vi "Find Hynix Spec.vi"(8 "error in":errorcluster) -> (0 "error out":errorcluster)   [LabVIEW 2020]
uses:
  Controls/Comm_Hynix Spec.ctl
  Controls/Cmd_File path.ctl
  <vilib>/Utility/sysdir.llb/System Directory Type.ctl
  Controls/Cmd_File Type.ctl
  <vilib>/Utility/NIReport.llb/Report Type.ctl
  Public/Polymorph/ini Ctrl_Str.vi
  Public/Polymorph/ini Ctrl_Var.vi
  <vilib>/security/Message Digest/API/Instances/File/SHA-256 File Checksum.vi
  <vilib>/addons/_office/excel.llb/Excel Get Data ([str]).vi
  <vilib>/Utility/NIReport.llb/NI_report.lvclass
  <vilib>/Utility/NIReport.llb/NI_ReportGenerationCore.lvlib
  <vilib>/addons/_office/NI_ReportGenerationToolkit.lvlib
  <vilib>/Utility/NIReport.llb/Excel/NI_Excel.lvclass
  <vilib>/security/Message Digest/API/NI_Message Digest API.lvlib
  <vilib>/addons/database/NI_Database_API.lvlib
panel:
  out "Status":string
  in  "파일 경로":path
  in  "팀":bool
  in  "모델":bool
  in  "제조사":bool
  in  "기기명":bool
  in  "Team SPEC":i32(listbox)
  in  "확인 버튼":bool
  in  "프로세스 정지 버튼":bool
  out "SPEC":string[][](table)
  in  "등록번호":string
  out "digest":string caption="요약"
  out "data":string[][](array[string])
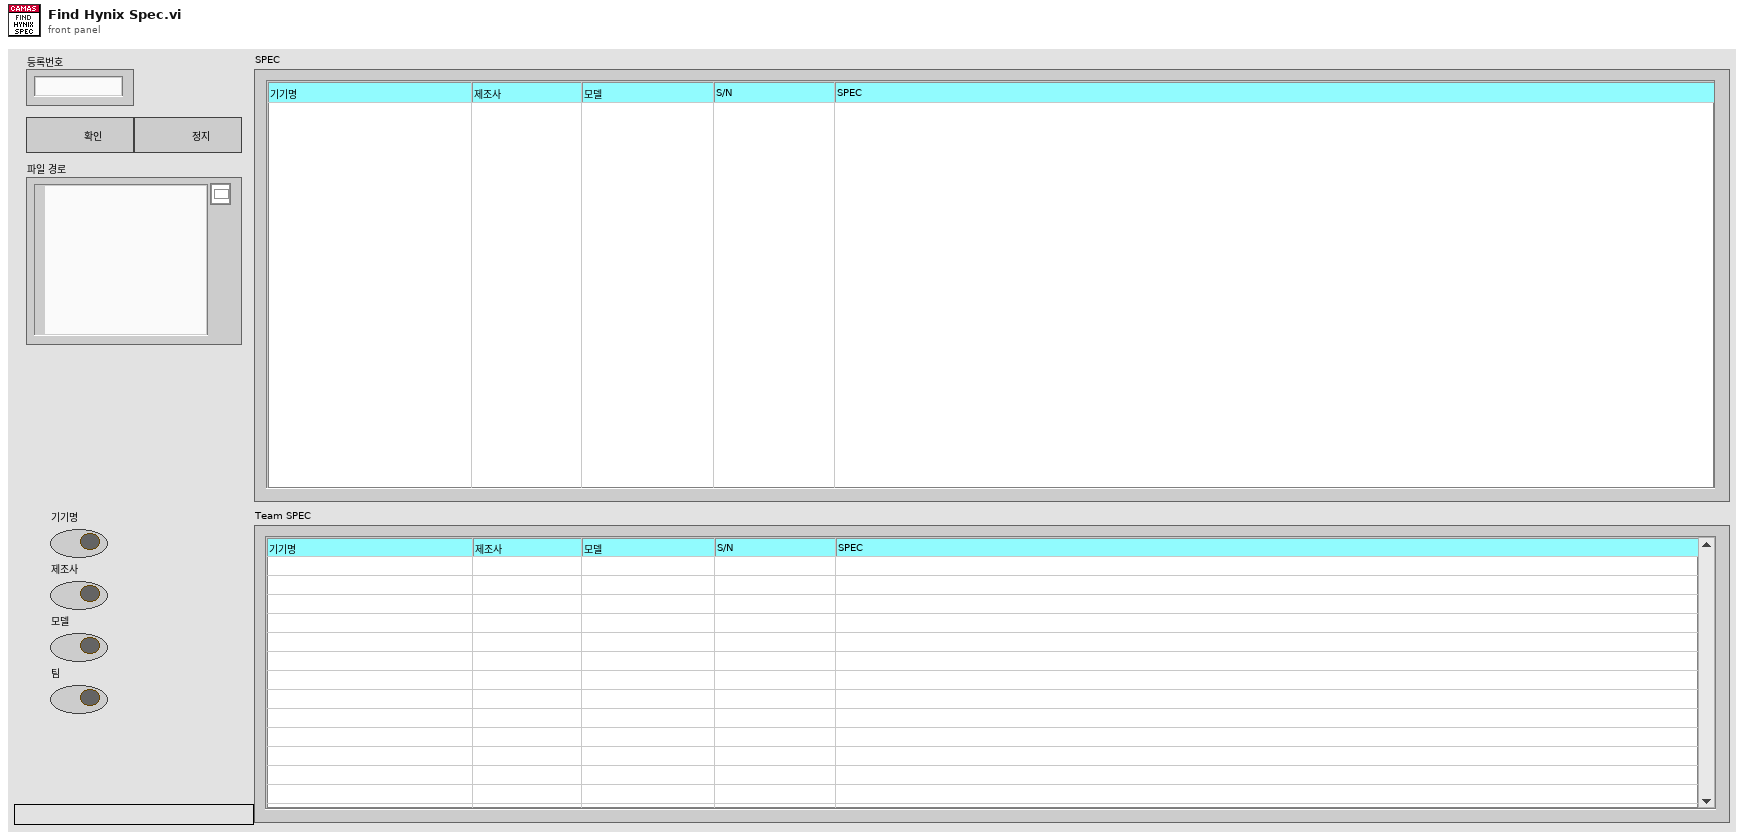
[diagram p1: front panel]
types:
  T1 = typedef "Comm_Hynix Spec.ctl" = enum16{"Initialize", "event", "File Open", "Find Spec", "Team Spec Open", "Error", "Exit"}
  T2 = typedef "Cmd_File Type.ctl" = enum16{"엑셀", "엑셀(2003)", "텍스트", "설정", "2진", "VI", "CSV", "LOG", "폴더"}
  T3 = typedef "Cmd_File path.ctl" = enum16{"에러로그", "데이터파일경로", "성적서원본", "지난성적서", "Data Files", "경로생성", "Updater", "Template", "설정파일경로", "FTP Upload", "Update 경로", "어플리케이션"}
  T4 = typedef "System Directory Type.ctl" = i32
  T5 = enum16{"open", "replace", "create", "open or create", "replace or create", "replace or create with confirmation"}
  T6 = typedef "NI_ReportGenerationCore.lvlib/Report Type.ctl" = enum16{"HTML", "Word", "Excel"}
  T7 = enum16{"maximized", "minimized", "normal", "no change"}
  T8 = cluster{"position (excel)":cluster{"row":i32, "column":i32}, "name (excel)":string, "bookmark (word)":string}
  T9 = typedef "NI_Database_API.lvlib/Conn ObjectReference.ctl" = refnum<k1>
  T10 = enum32{"invalid app kind", "Development System", "Run Time System", "Student Edition", "Embedded LabVIEW", "Evaluation", "Custom"}
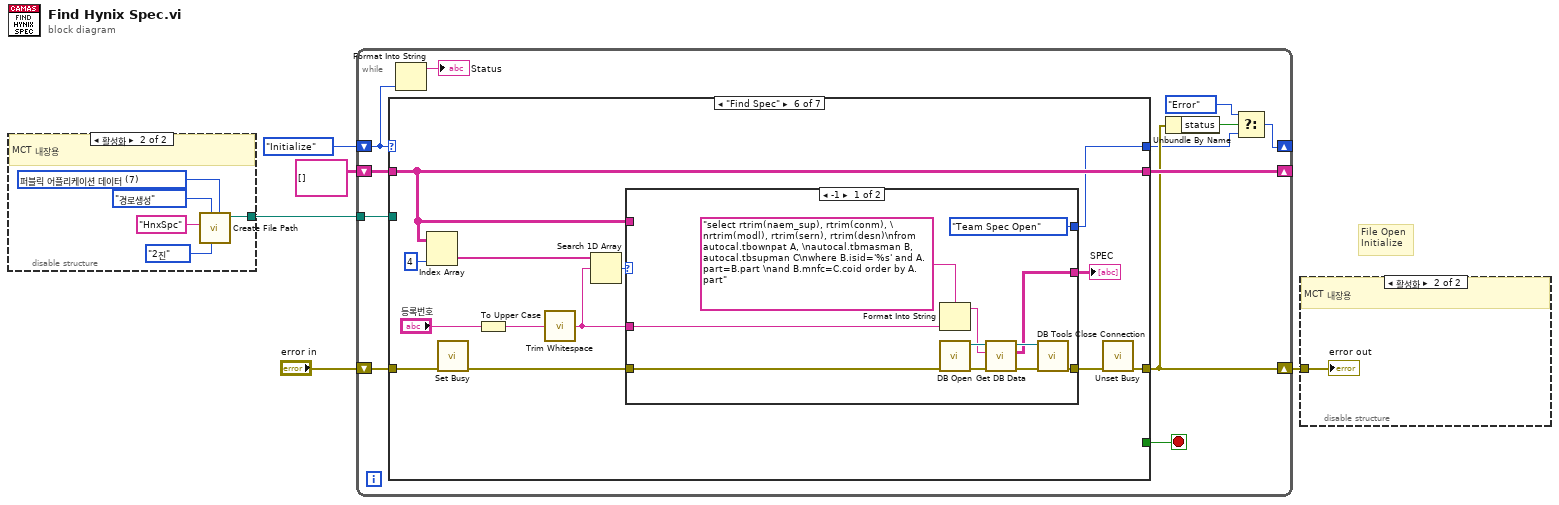
[diagram p0: block diagram]
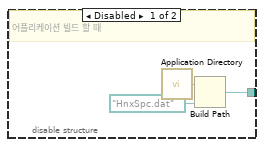
[diagram p2: hidden frame]
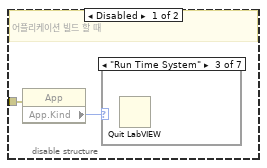
[diagram p3: hidden frame]
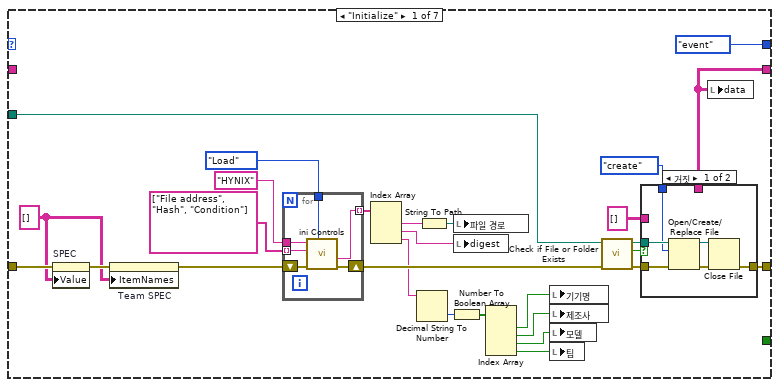
[diagram p10: hidden frame]
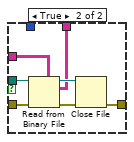
[diagram p11: hidden frame]
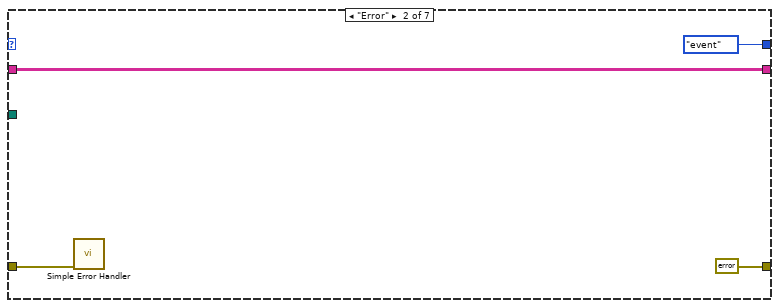
[diagram p12: hidden frame]
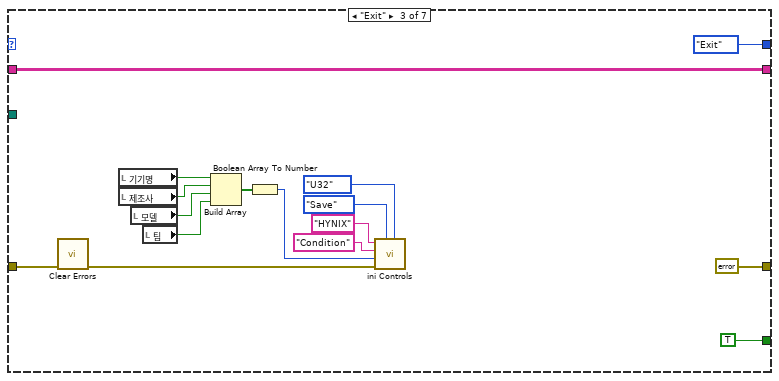
[diagram p13: hidden frame]
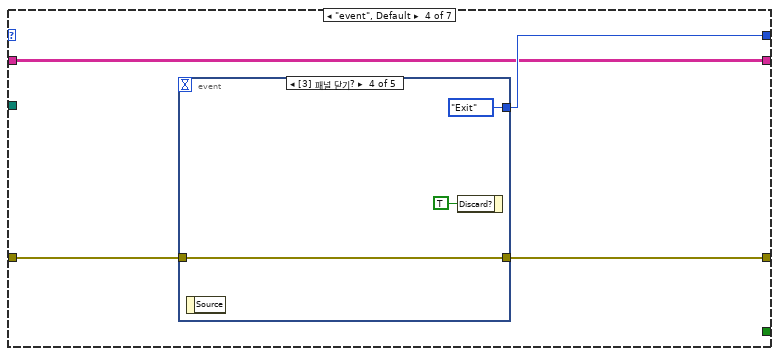
[diagram p14: hidden frame]
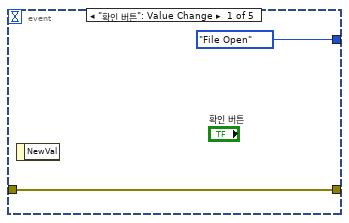
[diagram p15: hidden frame]
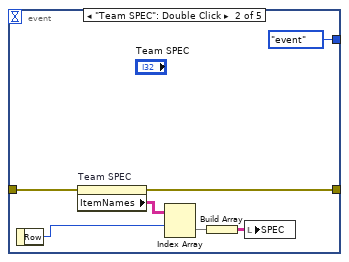
[diagram p16: hidden frame]
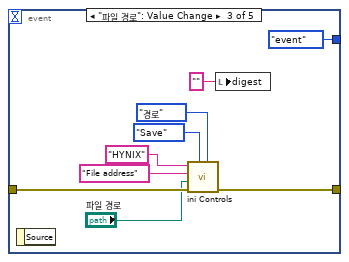
[diagram p17: hidden frame]
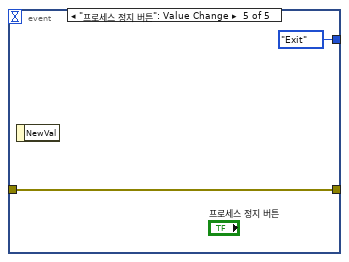
[diagram p18: hidden frame]
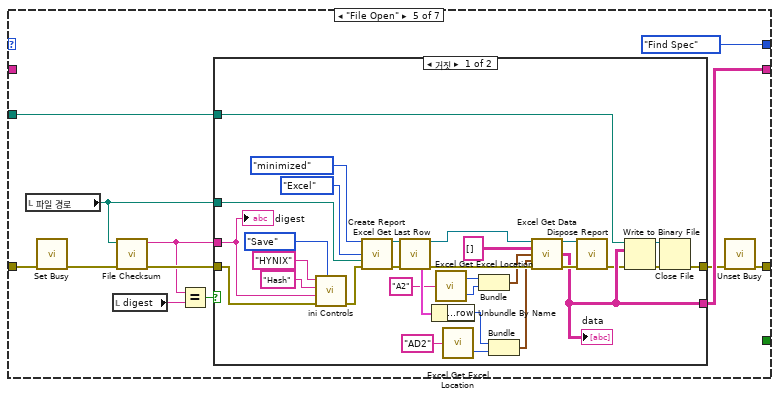
[diagram p19: hidden frame]
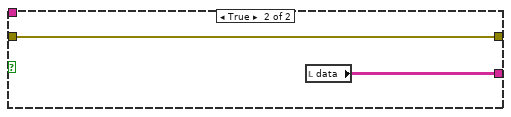
[diagram p20: hidden frame]
diagram:
  # "File Open\nInitialize"
  n1 = disable-structure shown="활성화" {
    disable-tunnel: [w6 w13] -> w1
    frame Disabled {
      # "어플리케이션 빌드 할 때"
      n2 = call <vilib>:"Application Directory.vi"() -> ("Application Directory"=w8:path)
      n3 = Build Path(base path=w8, name or relative path=path "HnxSpc.dat" ("이름 또는 상대 경로")) -> (appended path=w6:path)
    }
    frame Enabled {
      w11 = T4 7 items=["사용자 홈"=0, "사용자 데스크탑"=1, "사용자 문서"=2, "사용자 어플리케이션 데이터"=3, "사용자 환경"=4, "사용자 임시"=5, "퍼블릭 문서"=6, "퍼블릭 어플리케이션 데이터"=7, "퍼블릭 환경"=8, "퍼블릭 캐시"=13, "시스템 코어 라이브러리"=9, "시스템 설치된 라이브러리"=10, "어플리케이션 파일"=11, "부팅 볼륨 루트"=12] ("system directory type")
      # "MCT 내장용"
      n4 = call "Create File Path.vi"("system directory type"=w11, "파일타입"=Cmd_File_Type."2진", "항목"=Cmd_File_path."경로생성", "문자열 in"="HnxSpc" ("cell's name")) -> ("파일경로"=w13:path)  [unwired: 4 in, 3 out]
    }
  }
  n5 = while {
    shift-right: [w17] -> _
    shift-left: Comm_Hynix_Spec."Initialize" -> [w22]
    shift-right: [w24] -> _
    shift-left: string[][] [] ("data") -> [w25]
    shift-right: [w20] -> w4
    shift-left: "error in" -> [w23]
    tunnel: w1 -> [w15]
    stop <- w14 stop-if-true
    n6 = case shown="\"Find Spec\"" w22 {
      tunnel: [Comm_Hynix_Spec."event" Comm_Hynix_Spec."event" Comm_Hynix_Spec."Exit" w96 Comm_Hynix_Spec."Find Spec" w171 Comm_Hynix_Spec."event"] -> w18
      tunnel: w25 -> [_ w76 w92 w95 _ w173 w215]
      tunnel: [w35 w76 w92 w95 w127 w173 w215] -> w24
      tunnel: w23 -> [w52 w73 w89 w94 w126 w169 w211]
      tunnel: [w41 errorcluster {"status"=FALSE, "code"=0, "source"=""} ("에러 출력") errorcluster {"status"=FALSE, "code"=0, "source"=""} ("에러 출력") w93 w122 w166 w206] -> w20
      tunnel: w15 -> [w33 _ _ _ w120 _ _]
      tunnel: [_ _ TRUE _ _ _ _] -> w14
      frame "Initialize" {
        w50 = string[][] [] ("SPEC")
        n7 = property on="SPEC" class="Tbl (엄격한)"(error in=w52, "Value"=w50) -> (error out=w51:errorcluster)  [unwired: 1 in, 1 out]
        n8 = property on="Team SPEC" class="MCListbox (엄격한)"(error in=w51, "ItemNames"=w50) -> (error out=w49:errorcluster)  [unwired: 1 in, 1 out]
        n9 = for {
          tunnel: enum16{"Save", "Load"}."Load" ("Select") -> [w71]
          tunnel: string[] ["File address", "Hash", "Condition"] -> [w70] mode=indexing
          shift-right: [w69] -> w39
          shift-left: w49 -> [w72]
          tunnel: "HYNIX" ("섹션") -> [w68]
          tunnel: [w67] -> w44 mode=indexing
          n10 = call-poly "ini Controls.vi"("Select"=w71, "에러 입력"=w72, "키"=w70, "섹션"=w68) -> ("에러 출력"=w69:errorcluster, "값"=w67:string)  [unwired: 5 in, 1 out]
        }
        n11 = Index Array(array=w44) -> (element #1=w43:string, element #2=w42:string, element #3=w32:string)  [unwired: 3 in]
        n12 = Decimal String To Number(string=w32) -> (number=w31:i32)  [unwired: 2 in, 1 out]
        n13 = String To Path(string=w43) -> (path=w47:path)
        n14 = Number To Boolean Array(number=w31) -> (Boolean array=w30:bool[])
        n15 = local write "파일 경로"(w47) -> ()
        n16 = local write "digest"(w42) -> ()
        n17 = Index Array(array=w30) -> (element #1=w29:bool, element #2=w27:bool, element #3=w26:bool, element #4=w28:bool)  [unwired: 4 in]
        n18 = local write "기기명"(w29) -> ()
        n19 = local write "제조사"(w27) -> ()
        n20 = local write "모델"(w26) -> ()
        n21 = local write "팀"(w28) -> ()
        n22 = call <vilib>:"Check if File or Folder Exists.vi"("error in (no error)"=w39, "path"=w33) -> ("error out"=w38:errorcluster, "file or folder exists?"=w40:bool, "dup path"=w37:path)  [unwired: 7 in]
        n23 = case shown="거짓" w40 {
          tunnel: w38 -> [w59 w66]
          tunnel: w37 -> [w58 w65]
          tunnel: [w55 w62] -> w41
          tunnel: string[][] [] ("SPEC") -> [_ w61]
          tunnel: [_ w60] -> w35
          tunnel: T5."create" ("동작(0:open)") -> [w54 _]
          frame False {
            n24 = Open/Create/Replace File(file path (use dialog)=w58, error in=w59, operation (0:open)=w54) -> (refnum out=w57:refnum<file>, error out=w56:errorcluster)  [unwired: 3 in, 1 out]
            n25 = Close File(refnum=w57, error in=w56) -> (error out=w55:errorcluster)  [unwired: 1 out]
          }
          frame True {
            n26 = Read from Binary File(5:w61, 8:w66, 11:w65) -> (0:w64:errorcluster, 2:w60:string[][], 3:w63:refnum<file>)  [unwired: 3 in, 1 out]
            n27 = Close File(refnum=w63, error in=w64) -> (error out=w62:errorcluster)  [unwired: 1 out]
          }
        }
        n28 = local write "data"(w35) -> ()
      }
      frame "Error" {
        n29 = call <vilib>:"Simple Error Handler.vi"("error in (no error)"=w73) -> ()  [unwired: 4 in, 5 out]
      }
      frame "Exit" {
        n30 = call <vilib>:"Clear Errors.vi"("error in (no error)"=w89) -> ("error out"=w81:errorcluster)  [unwired: 5 in, 1 out]
        n31 = local read "기기명"() -> (w88:bool)
        n32 = local read "제조사"() -> (w87:bool)
        n33 = local read "모델"() -> (w85:bool)
        n34 = local read "팀"() -> (w86:bool)
        n35 = Build Array(w88, w87, w85, w86) -> (w80:bool[])
        n36 = Boolean Array To Number(Boolean array=w80) -> (number=w79:u32)
        n37 = call-poly "ini Controls.vi"("데이터타입"=enum16{"I16", "U32", "경로"}."U32", "Select"=enum16{"Save", "Load"}."Save", "에러 입력"=w81, "값"=w79, "키"="Condition", "섹션"="HYNIX") -> ()  [unwired: 3 in, 3 out]
      }
      frame "event", Default {
        n38 = event shown="[3] 패널 닫기?" {
          selector: _ -> [_ _ _ _ _]
          dyn-events: _ -> [_ _ _ _ _]
          timeout: _ -> [_ _ _ _ _]
          tunnel: [Comm_Hynix_Spec."File Open" Comm_Hynix_Spec."event" Comm_Hynix_Spec."event" Comm_Hynix_Spec."Exit" Comm_Hynix_Spec."Exit"] -> w96
          tunnel: w94 -> [w97 w105 w114 w117 w119]
          tunnel: [w97 w102 w113 w117 w119] -> w93
          event "확인 버튼": Value Change {
            n39 = event-data() -> ()  [unwired: 1 in, 1 out]
          }
          event "Team SPEC": Double Click {
            n40 = event-data() -> ("Row"=w103:i32)  [unwired: 1 in]
            n41 = property on="Team SPEC" class="MCListbox (엄격한)"(error in=w105) -> (error out=w102:errorcluster, "ItemNames"=w104:string[][])  [unwired: 1 in, 1 out]
            n42 = Index Array(array=w104, index (row)=w103) -> (element=w101:string[])  [unwired: 1 in]
            n43 = Build Array(w101) -> (w100:string[][])
            n44 = local write "SPEC"(w100) -> ()
          }
          event "파일 경로": Value Change {
            n45 = event-data() -> ()  [unwired: 1 in, 1 out]
            n46 = call-poly "ini Controls.vi"("데이터타입"=enum16{"I16", "U32", "경로"}."경로", "Select"=enum16{"Save", "Load"}."Save", "에러 입력"=w114, "값"="파일 경로", "키"="File address", "섹션"="HYNIX") -> ("에러 출력"=w113:errorcluster)  [unwired: 3 in, 2 out]
            n47 = local write "digest"("") -> ()
          }
          event Panel Close? {
            n48 = event-data() -> ()  [unwired: 1 in, 1 out]
            n49 = event-data("Discard?"=TRUE ("버림?")) -> ()  [unwired: 1 in, 1 out]
          }
          event "프로세스 정지 버튼": Value Change {
            n50 = event-data() -> ()  [unwired: 1 in, 1 out]
          }
        }
      }
      frame "File Open" {
        n51 = local read "파일 경로"() -> (w121:path)
        n52 = call <vilib>:"Set Busy.vi"("error in (no error)"=w126) -> ("error out"=w123:errorcluster)  [unwired: 9 in, 1 out]
        n53 = local read "digest"() -> (w131:string)
        n54 = call-poly <vilib>:"File Checksum.vi"("error in"=w123, "path"=w121) -> ("error out"=w129:errorcluster, "digest"=w128:string)  [unwired: 8 in]
        n55 = Equal?(x=w128, y=w131) -> (x = y?=w130:bool)
        n56 = case shown="거짓" w130 {
          tunnel: [w137 w164] -> w127
          tunnel: w121 -> [w144 _]
          tunnel: w129 -> [w140 w163]
          tunnel: w128 -> [w138 _]
          tunnel: [w136 w163] -> w125
          tunnel: w120 -> [w132 _]
          frame False {
            n57 = call-poly "ini Controls.vi"("Select"=enum16{"Save", "Load"}."Save", "에러 입력"=w140, "값"=w138, "키"="Hash", "섹션"="HYNIX") -> ("에러 출력"=w139:errorcluster)  [unwired: 4 in, 2 out]
            n58 = call <vilib>:"Create Report.vi"("window state (normal)"=T7."minimized", "report type"=Report_Type."Excel", "template (empty)"=w144, "error in (no error)"=w139) -> ("report out"=w159:refnum<class "NI_report.lvclass">, "error out"=w160:errorcluster)  [unwired: 10 in]
            n59 = call <vilib>:"Excel Get Last Row.vi"("report in"=w159, "error in (no error)"=w160) -> ("report out"=w158:refnum<class "NI_report.lvclass">, "MS Office parameters out"=w156:T8, "error out"=w157:errorcluster)  [unwired: 11 in]
            n60 = Unbundle By Name(w156) -> ("position (excel).row"=w148:i32)
            n61 = call <vilib>:"Excel Get Excel Location.vi"("cell's name"="A2") -> ("row"=w154:i32, "column"=w150:i32)
            n62 = call <vilib>:"Excel Get Excel Location.vi"("cell's name"="AD2") -> ("column"=w149:i32)  [unwired: 1 out]
            n63 = Bundle("row"=w154, "column"=w150) -> (w151:cluster{"row":i32, "column":i32})  [unwired: 1 in]
            n64 = Bundle("row"=w148, "column"=w149) -> (w147:cluster{"row":i32, "column":i32})  [unwired: 1 in]
            n65 = call-poly <vilib>:"Excel Get Data.vi"("report in"=w158, "data type"=string[][] [], "start (-1, -1)"=w151, "end (-1, -1)"=w147, "error in (no error)"=w157) -> ("report out"=w145:refnum<class "NI_report.lvclass">, "data"=w137:string[][], "error out"=w146:errorcluster)  [unwired: 8 in]
            "data" <- w137
            n66 = call-dynamic "Dispose Report.vi"("report in"=w145, "error in (no error)"=w146) -> ("error out"=w135:errorcluster)  [unwired: 13 in]
            n67 = Write to Binary File(file (use dialog)=w132, data=w137, error in=w135) -> (refnum out=w133:refnum<file>, error out=w134:errorcluster)  [unwired: 3 in, 1 out]
            n68 = Close File(refnum=w133, error in=w134) -> (error out=w136:errorcluster)  [unwired: 1 out]
            "digest" <- w138
          }
          frame True {
            n69 = local read "data"() -> (w164:string[][])
          }
        }
        n70 = call <vilib>:"Unset Busy.vi"("error in (no error)"=w125) -> ("error out"=w122:errorcluster)  [unwired: 10 in]
      }
      frame "Find Spec" {
        n71 = Index Array(array=w173, index (col)=4 ("비활성화된 인덱스 (열)")) -> (element=w177:string[])  [unwired: 1 in]
        n72 = call <vilib>:"Set Busy.vi"("error in (no error)"=w169) -> ("error out"=w167:errorcluster)  [unwired: 9 in, 1 out]
        n73 = To Upper Case(1:"등록번호") -> (0:w165:string)
        n74 = call <vilib>:"Trim Whitespace.vi"("string"=w165) -> ("trimmed string"=w170:string)  [unwired: 1 in]
        n75 = Search 1D Array(1D array=w177, element=w170) -> (index of element=w172:i32)  [unwired: 1 in]
        n76 = case shown="-1" w172 {
          selector: w172 -> [_ w191]
          tunnel: [w178 w196] -> w175
          tunnel: w173 -> [_ w192]
          tunnel: [Comm_Hynix_Spec."Team Spec Open" Comm_Hynix_Spec."event"] -> w171
          tunnel: w170 -> [w180 _]
          tunnel: w167 -> [w187 w189]
          tunnel: [w182 w189] -> w168
          frame -1 {
            n77 = Format Into String(format string="select rtrim(naem_sup), rtrim(conm), \nrtrim(modl), rtrim(sern), rtrim(desn)\nfrom autocal.tbownpat A, \nautocal.tbmasman B, autocal.tbsupman C\nwhere B.isid='%s' and A.part=B.part \nand B.mnfc=C.coid order by A.part" ("SQL query"), w180) -> (resulting string=w181:string)  [unwired: 2 in, 1 out]
            n78 = call "DB Open.vi"("에러 입력"=w187) -> ("에러 출력"=w185:errorcluster, "참조 번호 출력"=w186:T9)  [unwired: 9 in]
            n79 = call "Get DB Data.vi"("error in (no error)"=w185, "SQL query"=w181, "connection reference"=w186) -> ("error out"=w183:errorcluster, "Data"=w178:string[][], "connection reference"=w184:T9)  [unwired: 4 in, 2 out]
            n80 = call <vilib>:"DB Tools Close Connection.vi"("error in (no error)"=w183, "connection reference"=w184) -> ("error out"=w182:errorcluster)  [unwired: 5 in]
          }
          frame Default {
            n81 = Delete From Array(array=w192, index (row)=w191) -> (deleted portion=w201:string[])  [unwired: 2 in, 1 out]
            n82 = Index Array(array=w201, index #5=29 ("인덱스")) -> (element #1=w200:string, element #2=w199:string, element #3=w198:string, element #4=w195:string, element #5=w194:string)  [unwired: 4 in]
            n83 = Build Array(w200, w199, w198, w195, w194) -> (w197:string[])
            n84 = Build Array(w197) -> (w196:string[][])
          }
        }
        "SPEC" <- w175
        n85 = call <vilib>:"Unset Busy.vi"("error in (no error)"=w168) -> ("error out"=w166:errorcluster)  [unwired: 10 in]
      }
      frame "Team Spec Open" {
        n86 = local read "SPEC"() -> (w214:string[][])
        n87 = call <vilib>:"Set Busy.vi"("error in (no error)"=w211) -> ("error out"=w207:errorcluster)  [unwired: 9 in, 1 out]
        n88 = Index Array(array=w214, index (row)=0 ("인덱스 (행)")) -> (element=w212:string[])  [unwired: 1 in]
        n89 = Build Array("기기명", "제조사", "모델", "팀") -> (w208:bool[])
        n90 = for {
          tunnel: w215 -> [w230] mode=indexing
          tunnel: [w229] -> w209 mode=indexing if=w237
          tunnel: w212 -> [w239]
          tunnel: w208 -> [w228]
          n91 = Index Array(array=w230, index #4=10 ("인덱스")) -> (element #1=w223:string, element #2=w222:string, element #3=w221:string, element #4=w220:string)  [unwired: 3 in]
          n92 = Index Array(array=w239) -> (element #1=w227:string, element #2=w226:string, element #3=w225:string, element #5=w224:string)  [unwired: 5 in, 1 out]
          n93 = Build Array(w223, w222, w221, w220) -> (w219:string[])
          n94 = Build Array(w227, w226, w225, w224) -> (w218:string[])
          n95 = for {
            tunnel: w218 -> [w244] mode=indexing
            tunnel: w219 -> [w245] mode=indexing
            tunnel: w228 -> [w243] mode=indexing
            tunnel: [w240] -> w217 mode=indexing
            n96 = Equal?(x=w245, y=w244) -> (x = y?=w242:bool)
            n97 = Select(t=w242, s=w243, f=TRUE) -> (s? t:f=w240:bool)
          }
          n98 = And Array Elements(Boolean array=w217) -> (logical AND=w237:bool)
          n99 = Index Array(array=w230, index #5=29 ("인덱스")) -> (element #1=w236:string, element #2=w235:string, element #3=w234:string, element #4=w233:string, element #5=w232:string)  [unwired: 4 in]
          n100 = Build Array(w236, w235, w234, w233, w232) -> (w229:string[])
        }
        n101 = property on="Team SPEC" class="MCListbox (엄격한)"(error in=w207, "ItemNames"=w209) -> (error out=w210:errorcluster)  [unwired: 1 in, 1 out]
        n102 = call <vilib>:"Unset Busy.vi"("error in (no error)"=w210) -> ("error out"=w206:errorcluster)  [unwired: 10 in]
      }
    }
    n103 = Format Into String(w22) -> (resulting string=→"Status":string)  [unwired: 3 in, 1 out]
    n104 = Unbundle By Name(w20) -> ("status"=w19:bool)
    n105 = Select(t=Comm_Hynix_Spec."Error", s=w19, f=w18) -> (s? t:f=w17:T1)
  }
  n106 = disable-structure shown="활성화" {
    disable-tunnel: w4 -> [w247 w248]
    frame Disabled {
      # "어플리케이션 빌드 할 때"
      n107 = property class="App"(error in=w247) -> ("App.Kind"=w246:T10)  [unwired: 1 in, 2 out]
      n108 = case shown="\"Run Time System\"" w246 {
        frame "invalid app kind", Default {
        }
        frame "Development System" {
        }
        frame "Run Time System" {
          n109 = Quit LabVIEW() -> ()  [unwired: 1 in]
        }
        frame "Student Edition" {
        }
        frame "Embedded LabVIEW" {
        }
        frame "Evaluation" {
        }
        frame "Custom" {
        }
      }
    }
    frame Enabled {
      # "MCT 내장용"
      "error out" <- w248
    }
  }
